vi "VI Tree.vi"   [LabVIEW 2018, in "SF-10.lvlib"]
doc: "This is the instrument driver for the <INSTRUMENT NAME>. The VI Tree displays all the user-callable VIs of the instrument driver in an organized table."
uses:
  <instrlib>/SF-10/SF-10.lvlib
panel:
  # "(c) 2014 <Enter Company Name Here>.  ALL RIGHTS RESERVED."
  # "SEE DIAGRAM\nFOR VI TREE."
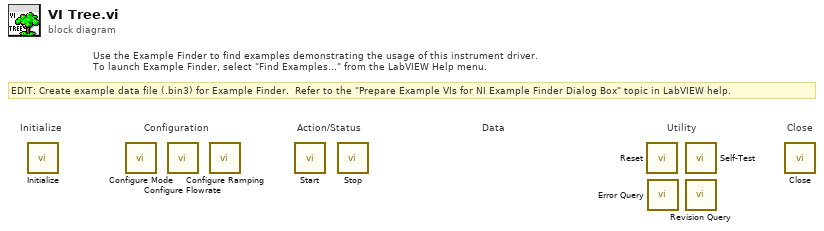
[diagram p0: block diagram]
diagram:
  # "EDIT: Create example data file (.bin3) for Example Finder.  Refer to the \"Prepare Example VIs for NI Example Finder Dialog Box\" topic in LabVIEW help."
  # "Use the Example Finder to find examples demonstrating the usage of this instrument driver.\nTo launch Example Finder, select \"Find Examples...\" from the LabVIEW Help menu."
  # "Configuration"
  # "Utility"
  # "Data"
  # "Action/Status"
  # "Close"
  # "Initialize"
  n1 = call <instrlib>:"Initialize.vi"() -> ()  [unwired: 10 in, 2 out]
  n2 = call <instrlib>:"Configure Mode.vi"() -> ()  [unwired: 12 in]
  n3 = call <instrlib>:"Configure Flowrate.vi"() -> ()  [unwired: 12 in]
  n4 = call <instrlib>:"Configure Ramping.vi"() -> ()  [unwired: 12 in]
  n5 = call <instrlib>:"Start.vi"() -> ()  [unwired: 12 in]
  n6 = call <instrlib>:"Stop.vi"() -> ()  [unwired: 12 in]
  n7 = call <instrlib>:"Reset.vi"() -> ()  [unwired: 10 in, 2 out]
  n8 = call <instrlib>:"Error Query.vi"() -> ()  [unwired: 8 in, 4 out]
  n9 = call <instrlib>:"Self-Test.vi"() -> ()  [unwired: 8 in, 4 out]
  n10 = call <instrlib>:"Revision Query.vi"() -> ()  [unwired: 8 in, 4 out]
  n11 = call <instrlib>:"Close.vi"() -> ()  [unwired: 11 in, 1 out]
